vi "ReadFromFile.vi"(3 "File paths":path[](array[path])) -> (0 "error out":errorcluster, 1 "Data Sets":T1[](array[typedef]) {"Settings"."Time" format="%<%H:%M\n%d/%m/%y>T"})   [LabVIEW 2014]
uses:
  <userlib>/CurtinCode/DataControl.ctl
  <userlib>/CurtinCode/SettingsControl.ctl
panel:
  out "text":string
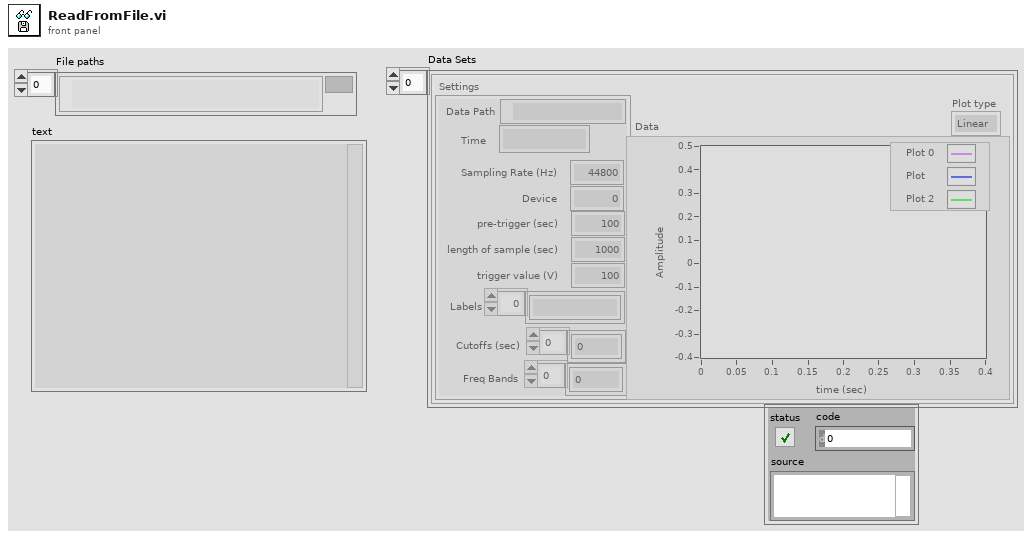
[diagram p1: front panel]
types:
  T1 = typedef "DataControl.ctl" = cluster{"Settings":T2, "Data":cluster{i32, dbl, "data":dbl[]}[], "Plot type":enum16{"Linear", "log"}}
  T2 = typedef "SettingsControl.ctl" = cluster{"Data Path":path, "Time":timestamp, "Sampling Rate (Hz)":u16, "Device":u16, "pre-trigger (sec)":dbl, "length of sample (sec)":dbl, "trigger value (V)":dbl, "Labels":string[], "Cutoffs (sec)":dbl[], "Freq Bands":dbl[]}
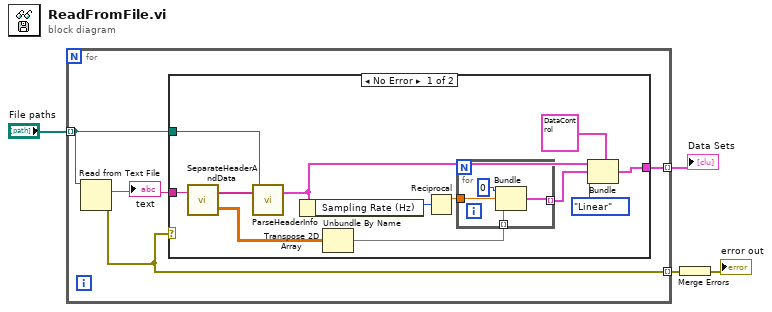
[diagram p0: block diagram]
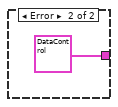
[diagram p2: hidden frame]
diagram:
  n1 = for {
    tunnel: "File paths" -> [w7] mode=indexing
    tunnel: [w5] -> w3 mode=indexing
    tunnel: [w6] -> w2 mode=indexing
    n2 = Read from Text File(file (use dialog)=w7) -> (text=w8:string, error out=w6:errorcluster)  [unwired: 3 in, 2 out]
    "text" <- w8
    n3 = case shown="No Error" w6 {
      tunnel: [w16 T1 {"Settings"={"Data Path"=path "", "Time"=timestamp(0 s since 1904-01-01), "Sampling Rate (Hz)"=44800, "Device"=0, "pre-trigger (sec)"=100.0, "length of sample (sec)"=1000.0, "trigger value (V)"=100.0, "Labels"=[], "Cutoffs (sec)"=[], "Freq Bands"=[]}, "Data"=[], "Plot type"=enum."Linear"} ("Data Set")] -> w5
      tunnel: w7 -> [w15 _]
      tunnel: w8 -> [w14 _]
      frame No Error {
        n4 = call <userlib>:"SeparateHeaderAndData.vi"("File Text"=w14) -> ("data"=w13:dbl[][], "Header Text"=w18:string[])  [unwired: 1 in]
        n5 = call <userlib>:"ParseHeaderInfo.vi"("Path In"=w15, "Header Lines"=w18) -> ("Parameters"=w17:T2)  [unwired: 1 in]
        n6 = Unbundle By Name(w17) -> ("Sampling Rate (Hz)"=w20:u16)
        n7 = Transpose 2D Array(2D array=w13) -> (transposed array=w9:dbl[][])
        n8 = Reciprocal(x=w20) -> (1/x=w19:dbl)
        n9 = for {
          tunnel: w19 -> [w23]
          tunnel: w9 -> [w22] mode=indexing
          tunnel: [w21] -> w10 mode=indexing
          n10 = Bundle(0, w23, w22) -> (w21:cluster{i32, dbl, dbl[]})  [unwired: 1 in]
        }
        n11 = Bundle(cluster=T1 {"Settings"={"Data Path"=path "", "Time"=timestamp(0 s since 1904-01-01), "Sampling Rate (Hz)"=44800, "Device"=0, "pre-trigger (sec)"=100.0, "length of sample (sec)"=1000.0, "trigger value (V)"=100.0, "Labels"=[], "Cutoffs (sec)"=[], "Freq Bands"=[]}, "Data"=[], "Plot type"=enum."Linear"} ("Data Set"), "Settings"=w17, "Data"=w10, "Plot type"=enum16{"Linear", "log"}."Linear") -> (w16:T1)
      }
      frame Error {
      }
    }
  }
  "Data Sets" <- w3
  n12 = Merge Errors(w2) -> (→"error out":errorcluster)
